vi "Recieve Lockin Data.vi"(8 "error in (no error)":errorcluster, 9 "Force read":bool, 10 "Points to read":i32, 11 "RP Lockin in":refnum<class "RP Transceiver.lvclass">) -> (0 "error out":errorcluster, 1 "Volatge X out":dbl[](array[numeric]), 2 "Frequency out":dbl[](array[numeric]), 3 "RP Lockin out":refnum<class "RP Transceiver.lvclass">, 4 "Starting edges":i32[](array[numeric]), 5 "Ending edges":i32[](array[numeric]), 6 "Volatge Y out":dbl[](array[numeric]))   [LabVIEW 2016, in "RP Transceiver.lvclass"]
uses:
  RP Transceiver.lvclass
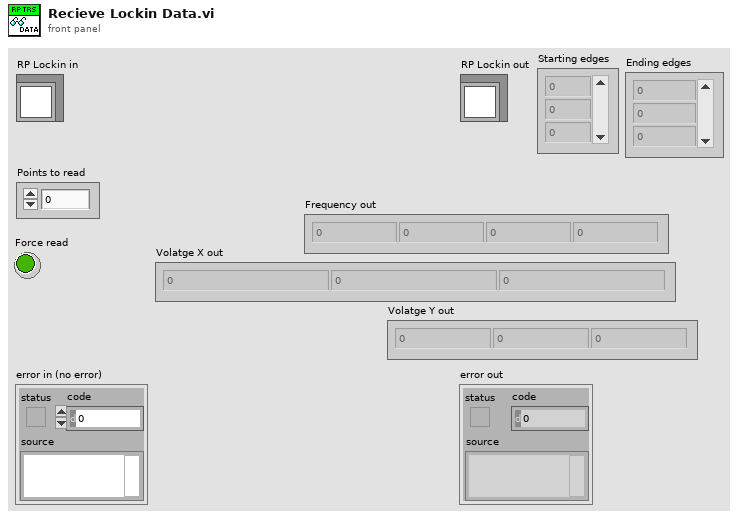
[diagram p1: front panel]
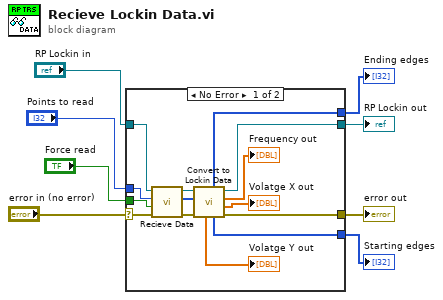
[diagram p0: block diagram]
diagram:
  n1 = case shown="No Error" "error in (no error)" {
    selector: "error in (no error)" -> [w22 w24]
    tunnel: [w19 w24] -> w7
    tunnel: [w20 w23] -> w5
    tunnel: "RP Lockin in" -> [w21 w23]
    tunnel: "Points to read" -> [w13 _]
    tunnel: "Force read" -> [w12 _]
    tunnel: [w11 _] -> w2
    tunnel: [w10 _] -> w1
    frame No Error {
      n2 = call-dynamic "Recieve Data.vi"("error in (no error)"=w22, "Force read"=w12, "Points to read"=w13, "RP Instrument in"=w21) -> ("error out"=w18:errorcluster, "Data out"=w17:i32[], "RP Instrument out"=w14:refnum<class "RP Transceiver.lvclass">)  [unwired: 5 in]
      n3 = call-dynamic "Convert to Lockin Data.vi"("error in (no error)"=w18, "Raw data"=w17, "RP Transceiver in"=w14) -> ("error out"=w19:errorcluster, "Volatge X out"=→"Volatge X out":dbl[], "Frequency out"=→"Frequency out":dbl[], "RP Transceiver out"=w20:refnum<class "RP Transceiver.lvclass">, "Starting edges"=w11:i32[], "Ending edges"=w10:i32[], "Volatge Y out"=→"Volatge Y out":dbl[])  [unwired: 2 in]
    }
    frame Error {
    }
  }
  "error out" <- w7
  "RP Lockin out" <- w5
  "Ending edges" <- w1
  "Starting edges" <- w2
